vi "PROXY_prepare_initialization_item_names.vi"(11 "all_config_info":T1) -> (2 "number_of_stations":i32, 3 "item_names":string[][](array[string]))   [LabVIEW 2020]
uses:
  ini/typedef/PROXY_all_config_info.ctl
  ini/typedef/PROXY_main_ini_file.ctl
  queues/typedef/PROXY_queue_refnums.ctl
  queues/typedef/STATION_queue_element.ctl
  STATION/ST_SQL_sequence_state.ctl
  _misc/AULocalize/SubVIs/Get Localized Phrase Compact Interface 0D.vi
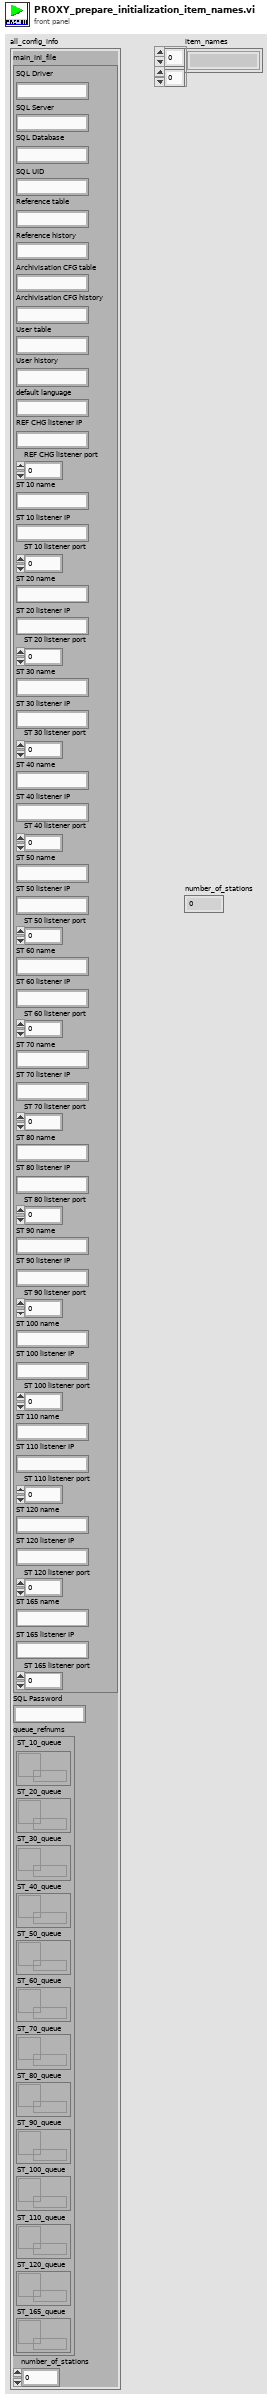
[diagram p1: front panel]
types:
  T1 = typedef "PROXY_all_config_info.ctl" = cluster{"main_ini_file":T2, "SQL Password":string, "queue_refnums":T3, "number_of_stations":i32}
  T2 = typedef "PROXY_main_ini_file.ctl" = cluster{"SQL Driver":string, "SQL Server":string, "SQL Database":string, "SQL UID":string, "Reference table":string, "Reference history":string, "Archivisation CFG table":string, "Archivisation CFG history":string, "User table":string, "User history":string, "default language":string, "REF CHG listener IP":string, "REF CHG listener port":u16, "ST 10 name":string, "ST 10 listener IP":string, "ST 10 listener port":u16, "ST 20 name":string, "ST 20 listener IP":string, "ST 20 listener port":u16, "ST 30 name":string, "ST 30 listener IP":string, "ST 30 listener port":u16, "ST 40 name":string, "ST 40 listener IP":string, "ST 40 listener port":u16, "ST 50 name":string, "ST 50 listener IP":string, "ST 50 listener port":u16, "ST 60 name":string, "ST 60 listener IP":string, "ST 60 listener port":u16, "ST 70 name":string, "ST 70 listener IP":string, "ST 70 listener port":u16, "ST 80 name":string, "ST 80 listener IP":string, "ST 80 listener port":u16, "ST 90 name":string, "ST 90 listener IP":string, "ST 90 listener port":u16, "ST 100 name":string, "ST 100 listener IP":string, "ST 100 listener port":u16, "ST 110 name":string, "ST 110 listener IP":string, "ST 110 listener port":u16, "ST 120 name":string, "ST 120 listener IP":string, "ST 120 listener port":u16, "ST 165 name":string, "ST 165 listener IP":string, "ST 165 listener port":u16}
  T3 = typedef "PROXY_queue_refnums.ctl" = cluster{"ST_10_queue":refnum<queue>, "ST_20_queue":refnum<queue>, "ST_30_queue":refnum<queue>, "ST_40_queue":refnum<queue>, "ST_50_queue":refnum<queue>, "ST_60_queue":refnum<queue>, "ST_70_queue":refnum<queue>, "ST_80_queue":refnum<queue>, "ST_90_queue":refnum<queue>, "ST_100_queue":refnum<queue>, "ST_110_queue":refnum<queue>, "ST_120_queue":refnum<queue>, "ST_165_queue":refnum<queue>}
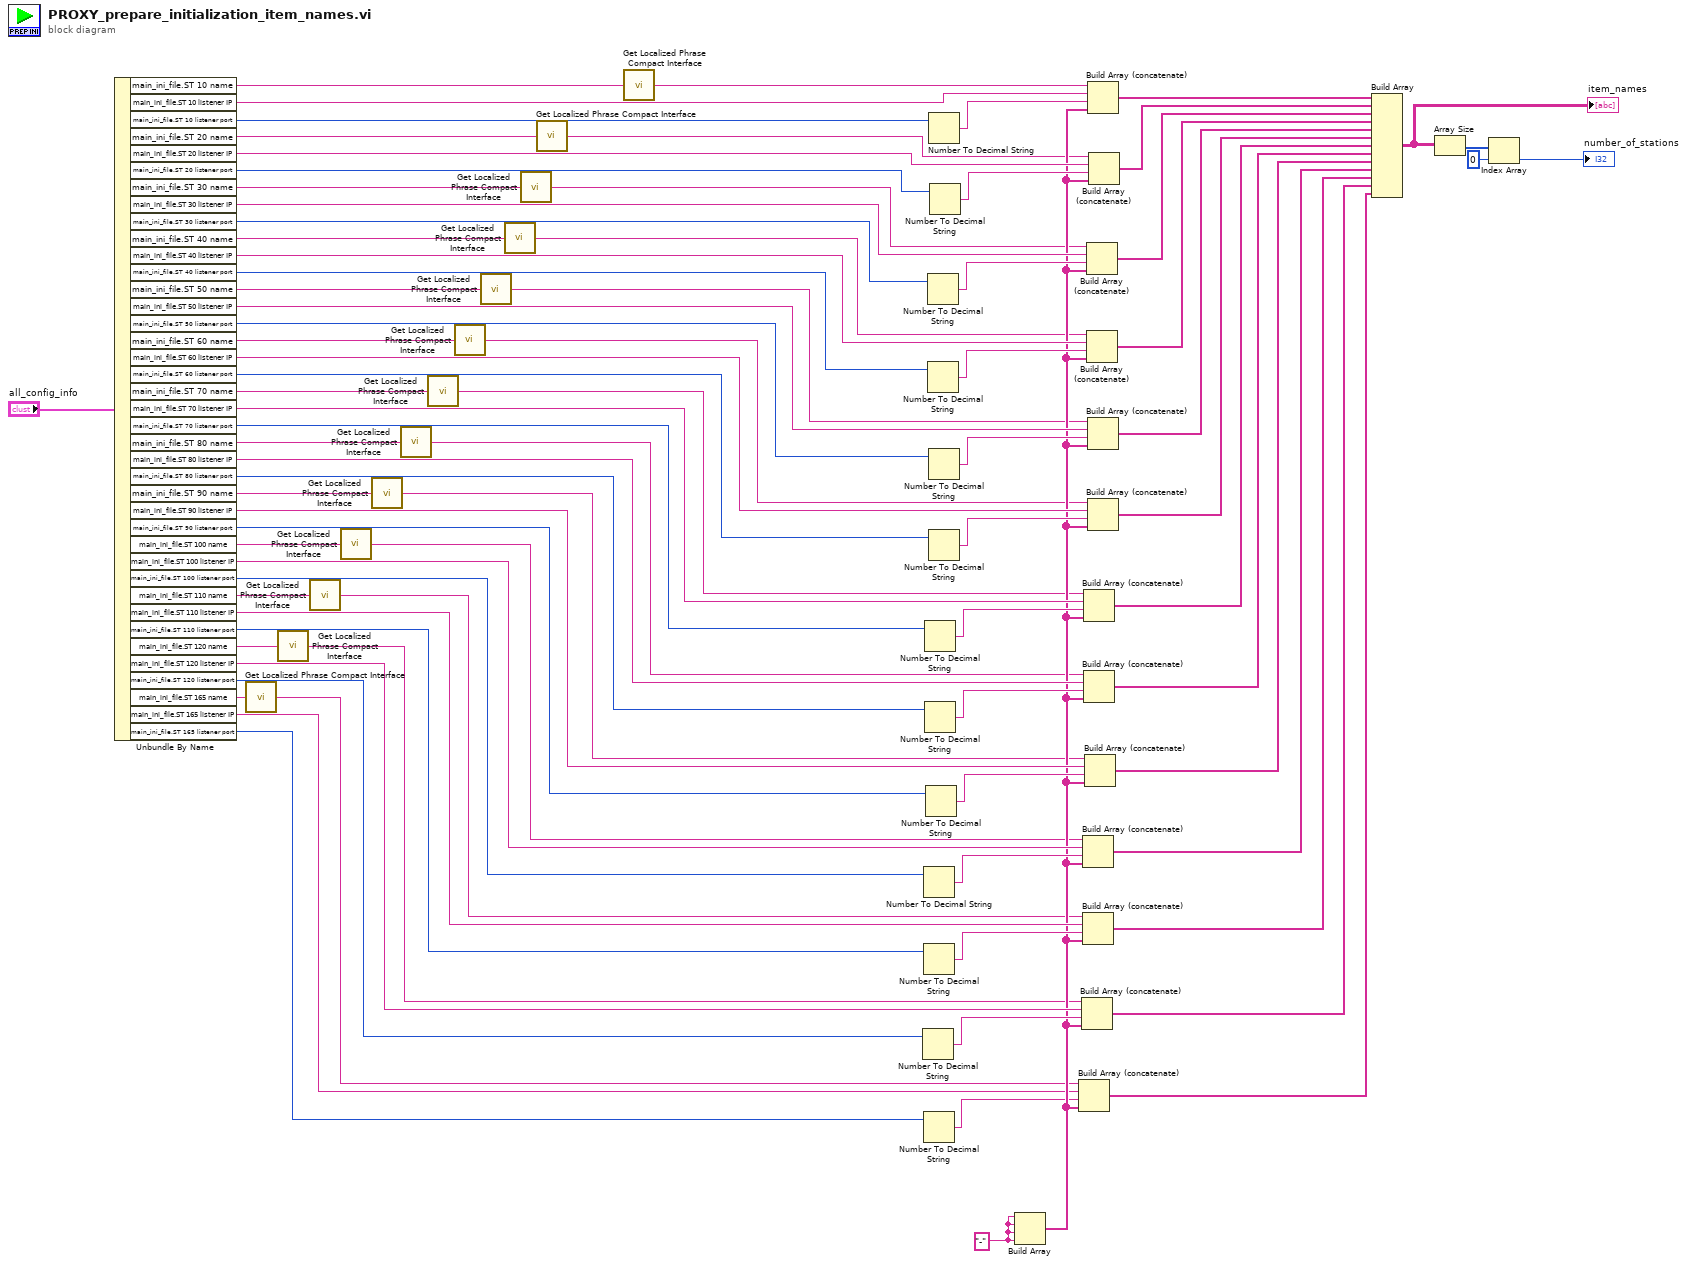
[diagram p0: block diagram]
diagram:
  w69 = "-"
  n1 = Unbundle By Name("all_config_info") -> ("main_ini_file.ST 10 name"=w81:string, "main_ini_file.ST 10 listener IP"=w82:string, "main_ini_file.ST 10 listener port"=w83:u16, "main_ini_file.ST 20 name"=w77:string, "main_ini_file.ST 20 listener IP"=w76:string, "main_ini_file.ST 20 listener port"=w75:u16, "main_ini_file.ST 30 name"=w72:string, "main_ini_file.ST 30 listener IP"=w71:string, "main_ini_file.ST 30 listener port"=w70:u16, "main_ini_file.ST 40 name"=w55:string, "main_ini_file.ST 40 listener IP"=w54:string, "main_ini_file.ST 40 listener port"=w53:u16, "main_ini_file.ST 50 name"=w52:string, "main_ini_file.ST 50 listener IP"=w51:string, "main_ini_file.ST 50 listener port"=w50:u16, "main_ini_file.ST 60 name"=w49:string, "main_ini_file.ST 60 listener IP"=w48:string, "main_ini_file.ST 60 listener port"=w47:u16, "main_ini_file.ST 70 name"=w46:string, "main_ini_file.ST 70 listener IP"=w45:string, "main_ini_file.ST 70 listener port"=w44:u16, "main_ini_file.ST 80 name"=w43:string, "main_ini_file.ST 80 listener IP"=w42:string, "main_ini_file.ST 80 listener port"=w41:u16, "main_ini_file.ST 90 name"=w40:string, "main_ini_file.ST 90 listener IP"=w39:string, "main_ini_file.ST 90 listener port"=w38:u16, "main_ini_file.ST 100 name"=w37:string, "main_ini_file.ST 100 listener IP"=w36:string, "main_ini_file.ST 100 listener port"=w35:u16, "main_ini_file.ST 110 name"=w34:string, "main_ini_file.ST 110 listener IP"=w33:string, "main_ini_file.ST 110 listener port"=w32:u16, "main_ini_file.ST 120 name"=w31:string, "main_ini_file.ST 120 listener IP"=w30:string, "main_ini_file.ST 120 listener port"=w29:u16, "main_ini_file.ST 165 name"=w16:string, "main_ini_file.ST 165 listener IP"=w15:string, "main_ini_file.ST 165 listener port"=w17:u16)
  n2 = call-poly "Get Localized Phrase Compact Interface.vi"("Key"=w16) -> ("Translated Phrase"=w1:string)
  n3 = call-poly "Get Localized Phrase Compact Interface.vi"("Key"=w31) -> ("Translated Phrase"=w2:string)
  n4 = call-poly "Get Localized Phrase Compact Interface.vi"("Key"=w34) -> ("Translated Phrase"=w3:string)
  n5 = call-poly "Get Localized Phrase Compact Interface.vi"("Key"=w37) -> ("Translated Phrase"=w4:string)
  n6 = call-poly "Get Localized Phrase Compact Interface.vi"("Key"=w40) -> ("Translated Phrase"=w5:string)
  n7 = call-poly "Get Localized Phrase Compact Interface.vi"("Key"=w43) -> ("Translated Phrase"=w6:string)
  n8 = call-poly "Get Localized Phrase Compact Interface.vi"("Key"=w46) -> ("Translated Phrase"=w7:string)
  n9 = call-poly "Get Localized Phrase Compact Interface.vi"("Key"=w49) -> ("Translated Phrase"=w8:string)
  n10 = call-poly "Get Localized Phrase Compact Interface.vi"("Key"=w52) -> ("Translated Phrase"=w9:string)
  n11 = call-poly "Get Localized Phrase Compact Interface.vi"("Key"=w55) -> ("Translated Phrase"=w10:string)
  n12 = call-poly "Get Localized Phrase Compact Interface.vi"("Key"=w72) -> ("Translated Phrase"=w11:string)
  n13 = call-poly "Get Localized Phrase Compact Interface.vi"("Key"=w77) -> ("Translated Phrase"=w12:string)
  n14 = call-poly "Get Localized Phrase Compact Interface.vi"("Key"=w81) -> ("Translated Phrase"=w13:string)
  n15 = Number To Decimal String(number=w29) -> (decimal integer string=w56:string)  [unwired: 1 in]
  n16 = Number To Decimal String(number=w35) -> (decimal integer string=w58:string)  [unwired: 1 in]
  n17 = Number To Decimal String(number=w32) -> (decimal integer string=w57:string)  [unwired: 1 in]
  n18 = Number To Decimal String(number=w17) -> (decimal integer string=w18:string)  [unwired: 1 in]
  n19 = Number To Decimal String(number=w44) -> (decimal integer string=w61:string)  [unwired: 1 in]
  n20 = Number To Decimal String(number=w41) -> (decimal integer string=w60:string)  [unwired: 1 in]
  n21 = Number To Decimal String(number=w38) -> (decimal integer string=w59:string)  [unwired: 1 in]
  n22 = Number To Decimal String(number=w70) -> (decimal integer string=w78:string)  [unwired: 1 in]
  n23 = Number To Decimal String(number=w53) -> (decimal integer string=w64:string)  [unwired: 1 in]
  n24 = Number To Decimal String(number=w83) -> (decimal integer string=w84:string)  [unwired: 1 in]
  n25 = Number To Decimal String(number=w50) -> (decimal integer string=w63:string)  [unwired: 1 in]
  n26 = Number To Decimal String(number=w47) -> (decimal integer string=w62:string)  [unwired: 1 in]
  n27 = Number To Decimal String(number=w75) -> (decimal integer string=w79:string)  [unwired: 1 in]
  n28 = Build Array(w69, w69, w69, w69) -> (w19:string[])
  n29 = Build Array (concatenate)(w1, w15, w18, w19) -> (w14:string[])
  n30 = Build Array (concatenate)(w2, w30, w56, w19) -> (w20:string[])
  n31 = Build Array (concatenate)(w4, w36, w58, w19) -> (w22:string[])
  n32 = Build Array (concatenate)(w3, w33, w57, w19) -> (w21:string[])
  n33 = Build Array (concatenate)(w7, w45, w61, w19) -> (w25:string[])
  n34 = Build Array (concatenate)(w6, w42, w60, w19) -> (w24:string[])
  n35 = Build Array (concatenate)(w5, w39, w59, w19) -> (w23:string[])
  n36 = Build Array (concatenate)(w11, w71, w78, w19) -> (w73:string[])
  n37 = Build Array (concatenate)(w10, w54, w64, w19) -> (w28:string[])
  n38 = Build Array (concatenate)(w13, w82, w84, w19) -> (w85:string[])
  n39 = Build Array (concatenate)(w9, w51, w63, w19) -> (w27:string[])
  n40 = Build Array (concatenate)(w8, w48, w62, w19) -> (w26:string[])
  n41 = Build Array (concatenate)(w12, w76, w79, w19) -> (w74:string[])
  n42 = Build Array(w85, w74, w73, w28, w27, w26, w25, w24, w23, w22, w21, w20, w14) -> (w68:string[][])
  "item_names" <- w68
  n43 = Array Size(array=w68) -> (size(s)=w67:i32[])
  n44 = Index Array(array=w67, index=0) -> (element=→"number_of_stations":i32)
